vi "Send Value Update.vi"(8 "error in (no error)":errorcluster, 9 "Value":variant, 10 "Datum Name":string, 11 "IViewModel in":refnum<class "IViewModel.lvclass">) -> (0 "error out":errorcluster)   [LabVIEW 2020, in "IViewModel.lvlib" / "IViewModel.lvclass"]
doc: "发送值更新"
uses:
  IViewModel.lvclass
  mva-core/Source/IObserver/IObserver/IObserver.lvclass/IObserver.ctl
  IViewModel.lvclass/IViewModel.ctl
  mva-core/Source/IMediator/PublishRequest/PublishRequest.lvclass/PublishRequest.ctl
  mva-core/Source/IMediator/IMediator Messages/Publish Msg/Publish Msg.lvclass/Publish Msg.ctl
  composed-af-messages/Source/RoundTripMessage/RoundTripMessage.lvclass/RoundTripMessage.ctl
  <vilib>/ActorFramework/Message Enqueuer/Message Enqueuer.lvclass/Message Enqueuer.ctl
  mva-core/Source/IMediator/IMediator Messages/Publish Msg/Send Pre-Addressed Publish.vi
  mva-core/Source/IObserver/IObserver/Read Unique ID.vi
  mva-core/Source/IMediator/PublishRequest/Pack Publish Request.vi
  composed-af-messages/Source/RoundTripMessage/Return Round-Trip Message.vi
  <vilib>/ActorFramework/Message Enqueuer/Enqueue.vi
  mva-core/Source/IMediator/IMediator Messages/Publish Msg/Publish Msg.lvclass
  composed-af-messages/Source/RoundTripMessage/RoundTripMessage.lvclass
  C:/Program Files/National Instruments/LabVIEW 2020/vi.lib/ActorFramework/Message/Message.lvclass
  <vilib>/Utility/error.llb/Error Cluster From Error Code.vi
  <vilib>/ActorFramework/Message Priority Queue/Priority Enqueue.vi
  mva-core/Source/IMediator/PublishRequest/PublishRequest.lvclass
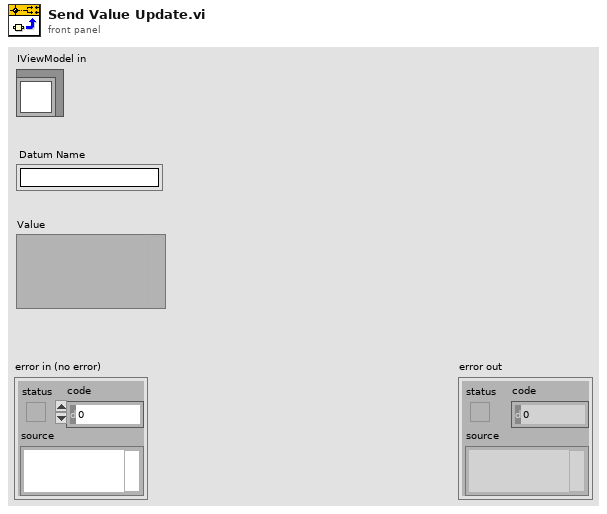
[diagram p1: front panel]
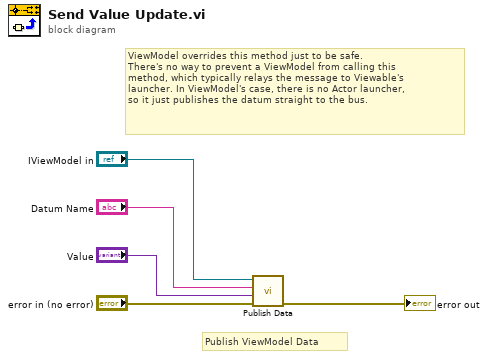
[diagram p0: block diagram]
diagram:
  # "ViewModel overrides this method just to be safe.\nThere's no way to prevent a ViewModel from calling this\nmethod, which typically relays the message to Viewable's\nlauncher. In ViewModel's case, there is no Actor launcher,\nso it just publishes the datum straight to the bus."
  # "Publish ViewModel Data"
  n1 = call "Publish Data.vi"("error in (no error)"="error in (no error)", "Data to Publish"="Value", "Datum Name"="Datum Name", "IViewModel In"="IViewModel in") -> ("error out"=→"error out":errorcluster)  [unwired: 6 in, 1 out]
